vi "Table Load.vi"(8 "error in (no error)":errorcluster, 11 "Work No":refnum<vi>) -> ()   [LabVIEW 2019]
uses:
  Ctrl/Table Save.ctl
  <vilib>/Utility/xml.llb/Read From XML File(string).vi
  LLB/Commonly VI/Main Glb.vi
  <vilib>/Utility/xml.llb/Write to XML File(string).vi
  LLB/Commonly VI.lvlib
panel:
  out "NG數量":string
  out "良品數量":string
  out "工單號碼Table":cluster{"Table Control":string[][]}[](array[cluster])
  out "EnfMeasureTable":cluster{"Table Control":string[][]}[](array[cluster])
  in  "EnfMeasureTable 5":cluster{"Table Control":string[][]}[](array[cluster])
  out "EnfMeasureTable 3":cluster{"Table Control":string[][]}[](array[cluster])
  out "value":cluster{"Table Control":string[][]}[](array[cluster])
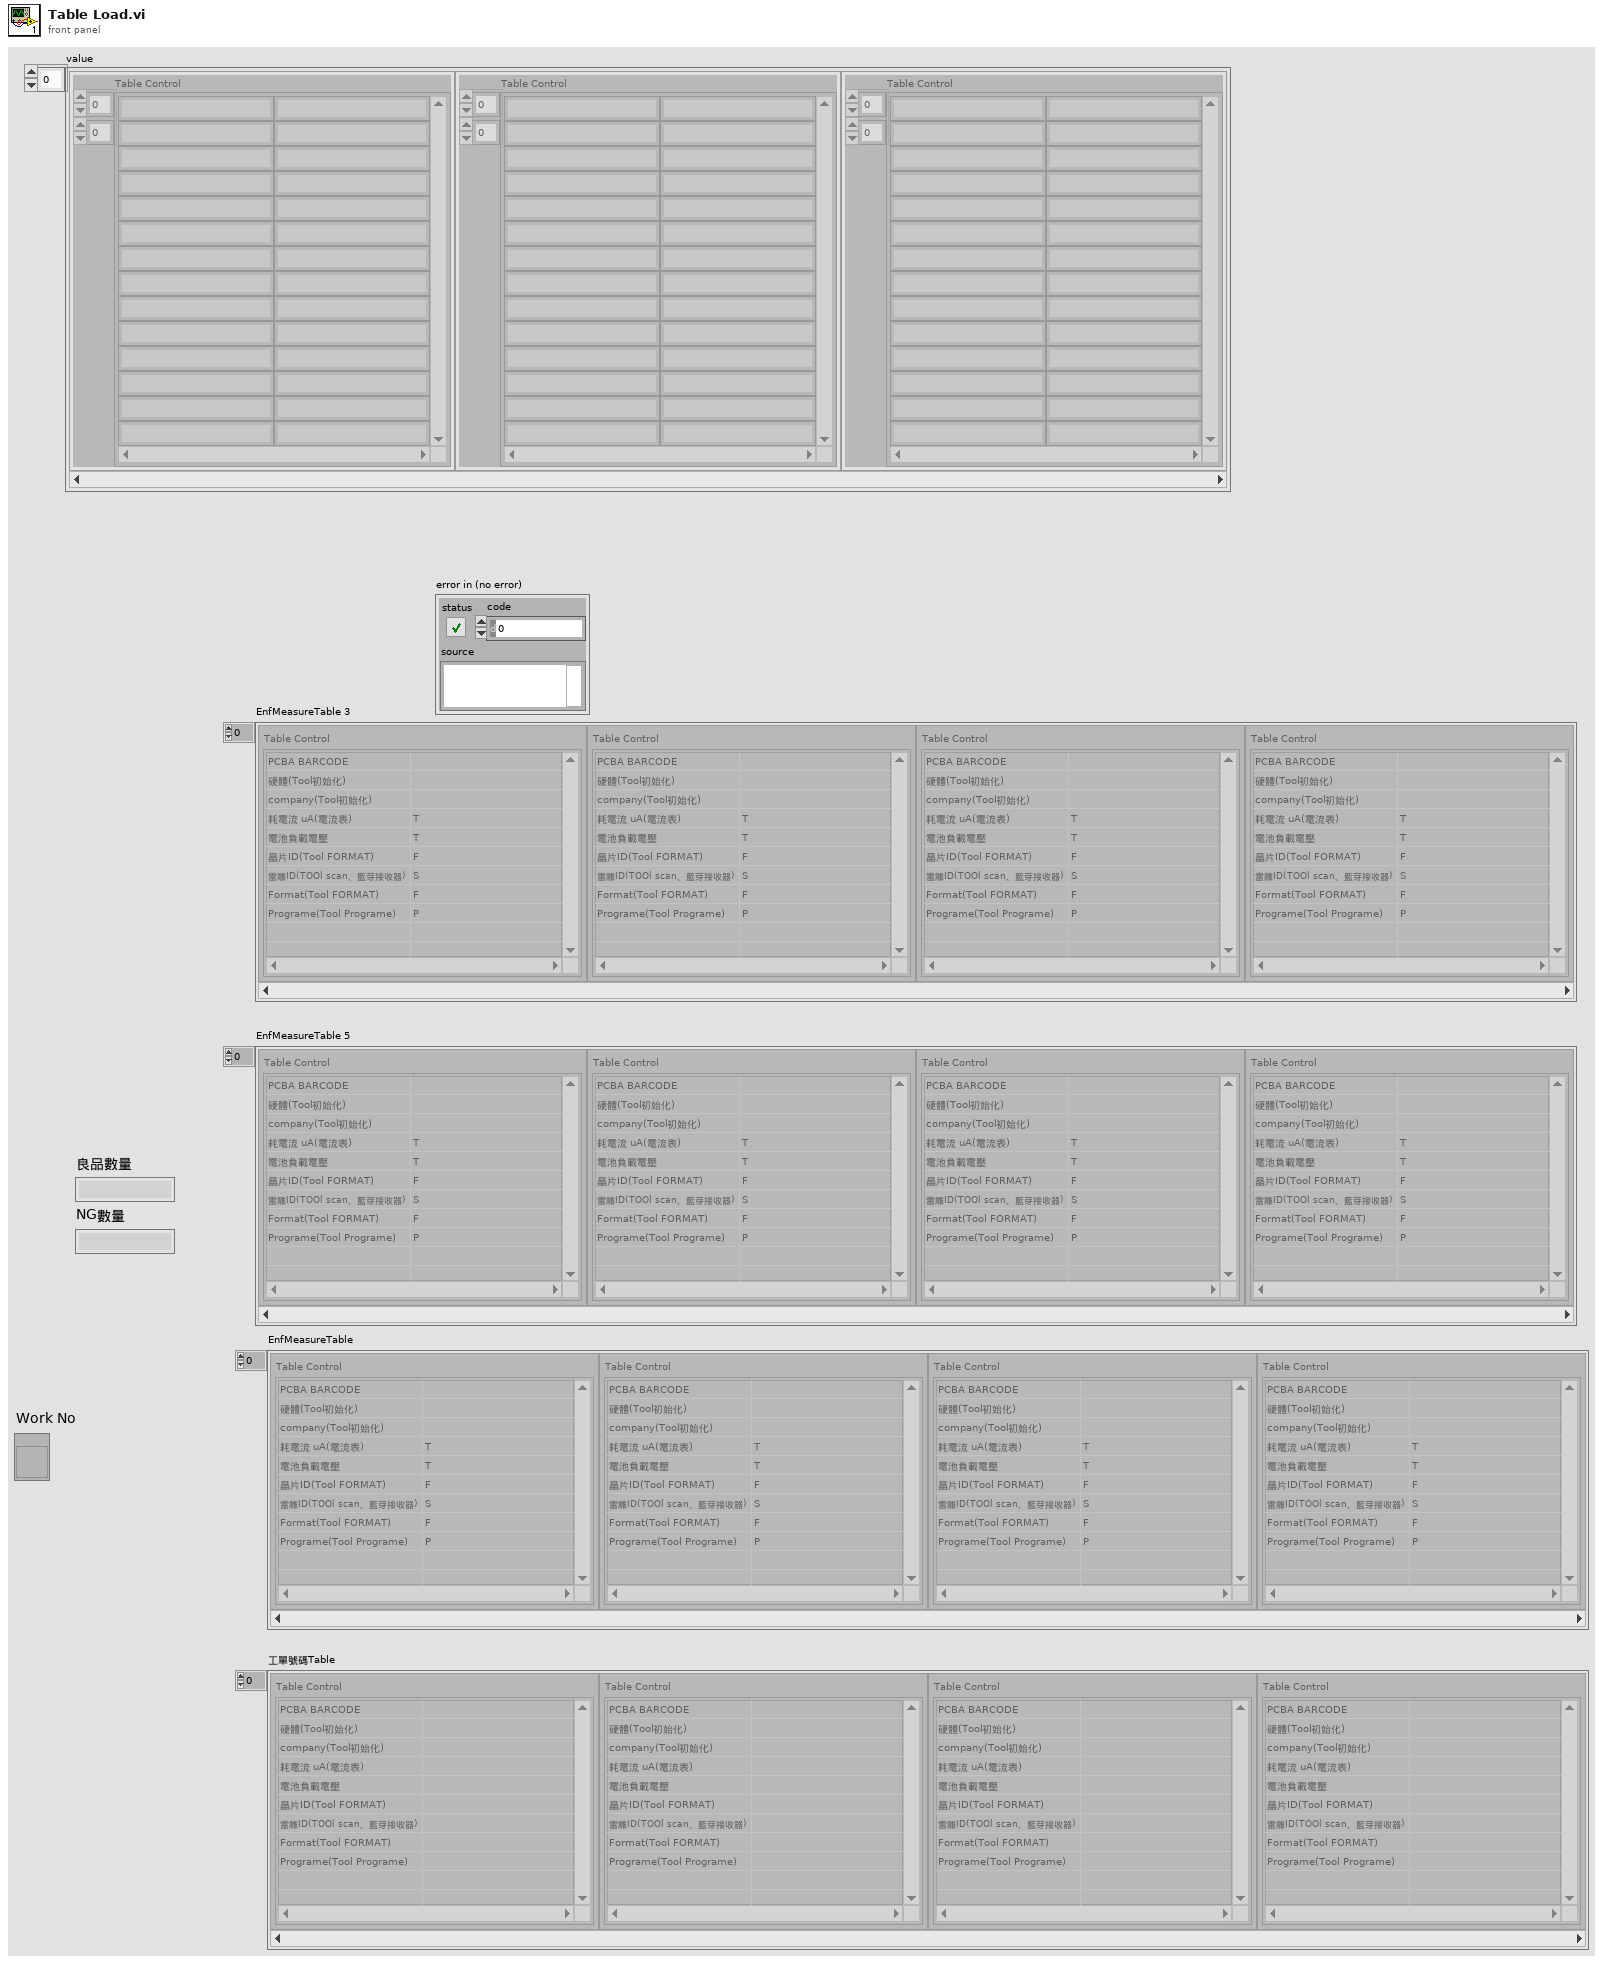
[diagram p1: front panel]
types:
  T1 = typedef "Table Save.ctl" = enum16{"initial", "Add", "Write", "Replace", "Delete", "REad", "RedTable", "Load"}
  T2 = typedef "工單號碼_Index.ctl" = enum16{"工單號碼", "產品料號", "品名", "作業員", "生產總數", "量品數量", "NG數量", "良率%"}
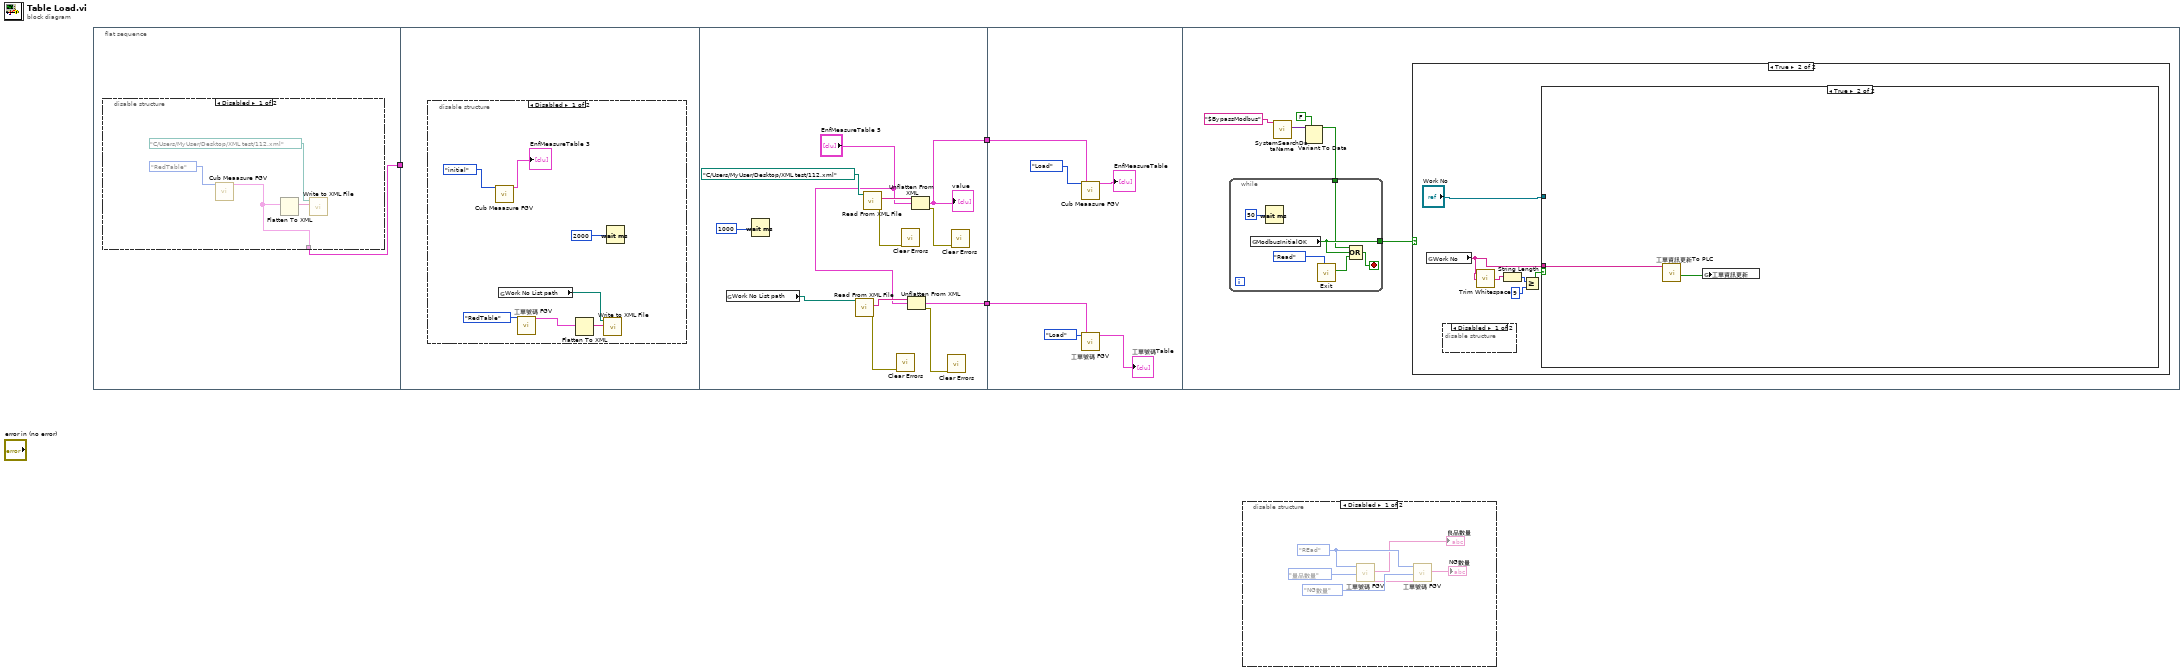
[diagram p0: block diagram]
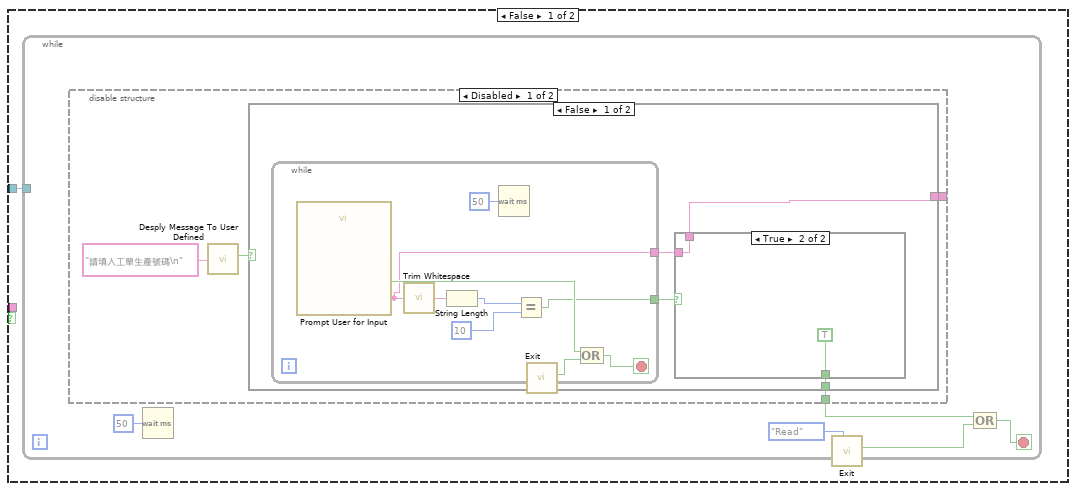
[diagram p6: hidden frame]
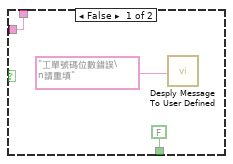
[diagram p7: hidden frame]
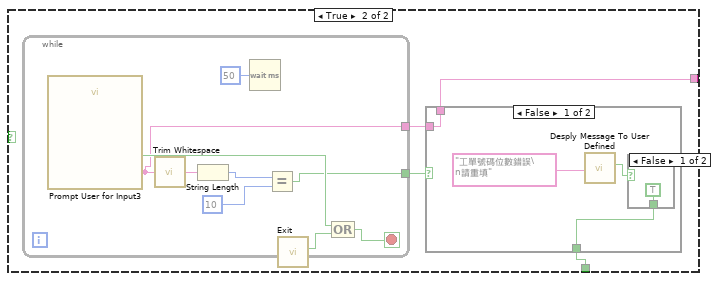
[diagram p8: hidden frame]
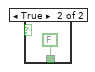
[diagram p9: hidden frame]
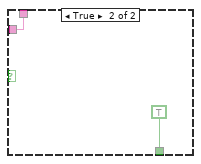
[diagram p10: hidden frame]
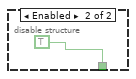
[diagram p11: hidden frame]
diagram:
  n1 = flat-sequence {
    tunnel: [w4] -> w3
    tunnel: w3 -> [_]
    tunnel: [w24] -> w2
    tunnel: [w18] -> w1
    tunnel: w2 -> [w31]
    tunnel: w1 -> [w29]
    frame #0 {
      n2 = disable-structure shown="Disabled" {
        disable-tunnel: [w5 _] -> w4
        frame Disabled {
          n3 = call "Cub Meaasure FGV.vi"("Action"=Table_Save."RedTable") -> ("Total Table"=w5:cluster{"Table Control":string[][]}[])  [unwired: 8 in, 6 out]
          n4 = Flatten To XML(anything=w5) -> (xml string=w8:string)
          n5 = call-poly <vilib>:"Write to XML File.vi"("XML Input"=w8, "XML File Path"=path "C:/Users/MyUser/Desktop/XML test/112.xml") -> ()  [unwired: 7 in, 3 out]
        }
        frame Enabled {
        }
      }
    }
    frame #1 {
      n6 = disable-structure shown="Disabled" {
        frame Disabled {
          n7 = call "Cub Meaasure FGV.vi"("Action"=Table_Save."initial") -> ("Total Table"=→"EnfMeasureTable 3":cluster{"Table Control":string[][]}[])  [unwired: 8 in, 6 out]
          n8 = global read "Main Glb.vi" "Work No List path"() -> (w12:path)
          n9 = call "工單號碼 FGV.vi"("Action"=Table_Save."RedTable") -> ("Total Table"=w10:cluster{"Table Control":string[][]}[])  [unwired: 11 in, 7 out]
          n10 = Flatten To XML(anything=w10) -> (xml string=w11:string)
          n11 = call-poly <vilib>:"Write to XML File.vi"("XML Input"=w11, "XML File Path"=w12) -> ()  [unwired: 7 in, 3 out]
          n12 = Wait (ms)(milliseconds to wait=2000) -> ()  [unwired: 1 out]
        }
        frame Enabled {
        }
      }
    }
    frame #2 {
      n13 = global read "Main Glb.vi" "Work No List path"() -> (w21:path)
      n14 = Wait (ms)(milliseconds to wait=1000) -> ()  [unwired: 1 out]
      n15 = call-poly <vilib>:"Read From XML File.vi"("XML File Path"=w21) -> ("error out"=w20:errorcluster, "XML Elements"=w19:string)  [unwired: 8 in, 1 out]
      n16 = call-poly <vilib>:"Read From XML File.vi"("XML File Path"=path "C:/Users/MyUser/Desktop/XML test/112.xml") -> ("error out"=w22:errorcluster, "XML Elements"=w27:string)  [unwired: 8 in, 1 out]
      n17 = call <vilib>:"Clear Errors.vi"("error in (no error)"=w20) -> ()  [unwired: 5 in, 2 out]
      n18 = call <vilib>:"Clear Errors.vi"("error in (no error)"=w22) -> ()  [unwired: 5 in, 2 out]
      n19 = Unflatten From XML(xml string=w19, type="EnfMeasureTable 5") -> (value=w18:cluster{"Table Control":string[][]}[], error out=w16:errorcluster)  [unwired: 1 in]
      n20 = Unflatten From XML(xml string=w27, type="EnfMeasureTable 5") -> (value=w24:cluster{"Table Control":string[][]}[], error out=w23:errorcluster)  [unwired: 1 in]
      "value" <- w24
      n21 = call <vilib>:"Clear Errors.vi"("error in (no error)"=w16) -> ()  [unwired: 5 in, 2 out]
      n22 = call <vilib>:"Clear Errors.vi"("error in (no error)"=w23) -> ()  [unwired: 5 in, 2 out]
    }
    frame #3 {
      n23 = call "Cub Meaasure FGV.vi"("Action"=Table_Save."Load", "Table Load"=w31) -> ("Total Table"=→"EnfMeasureTable":cluster{"Table Control":string[][]}[])  [unwired: 10 in, 7 out]
      n24 = call "工單號碼 FGV.vi"("Action"=Table_Save."Load", "Table Load"=w29) -> ("Total Table"=→"工單號碼Table":cluster{"Table Control":string[][]}[])  [unwired: 10 in, 7 out]
    }
    frame #4 {
      n25 = call "SystemSearchDataName.vi"("element"="$BypassModbus") -> ("variant"=w37:variant)  [unwired: 8 in, 2 out]
      n26 = Variant To Data(type=FALSE, Variant=w37) -> (data=w34:bool)  [unwired: 1 in, 1 out]
      n27 = while {
        tunnel: [w99] -> w38
        tunnel: w34 -> [w97]
        stop <- w100 stop-if-true
        n28 = global read "Main Glb.vi" "ModbusInitialOK"() -> (w99:bool)
        n29 = Wait (ms)(milliseconds to wait=50) -> ()  [unwired: 1 out]
        n30 = call "Exit.vi"("Enum"=enum16{"Initial", "Read", "Write"}."Read") -> ("ExitOut"=w101:bool)  [unwired: 10 in]
        n31 = Compound Arithmetic op=OR(w97, w99, w101) -> (w100:bool)
      }
      n32 = case shown="True" w38 {
        frame False {
        }
        frame True {
          n33 = global read "Main Glb.vi" "Work No"() -> (w40:string)
          n34 = disable-structure shown="Disabled" {
            frame Disabled {
            }
            frame Enabled {
            }
          }
          n35 = call <vilib>:"Trim Whitespace.vi"("string"=w40) -> ("trimmed string"=w39:string)  [unwired: 1 in]
          n36 = String Length(string=w39) -> (length=w44:i32)
          n37 = Greater Or Equal?(x=w44, y=9) -> (x >= y?=w42:bool)
          n38 = case shown="True" w42 {
            tunnel: w40 -> [_ w96]
            tunnel: "Work No" -> [w45 _]
            frame False {
              n39 = while {
                tunnel: w45 -> [_]
                stop <- w46 stop-if-true
                n40 = disable-structure shown="Disabled" {
                  disable-tunnel: [w52 TRUE] -> w49
                  disable-tunnel: [w51 _] -> _
                  frame Disabled {
                    n41 = call "Desply Message To User Defined.vi"("Message"="請填入工單生產號碼\n") -> ("關閉/Close"=w53:bool)  [unwired: 9 in, 1 out]
                    n42 = case shown="False" w53 {
                      tunnel: [w56 w74] -> w51
                      tunnel: [w55 w73] -> w52
                      frame False {
                        n43 = while {
                          tunnel: [w66] -> w58
                          tunnel: [w65] -> w57
                          stop <- w68 stop-if-true
                          n44 = call "Prompt User for Input"() -> ("Work No"=w65:string, "OK"=w67:bool)  [unwired: 17 in, 1 out]
                          n45 = call <vilib>:"Trim Whitespace.vi"("string"=w65) -> ("trimmed string"=w72:string)  [unwired: 1 in]
                          n46 = String Length(string=w72) -> (length=w71:i32)
                          n47 = Wait (ms)(milliseconds to wait=u32 50) -> ()  [unwired: 1 out]
                          n48 = Equal?(x=w71, y=10) -> (x = y?=w66:bool)
                          n49 = call "Exit.vi"() -> ("ExitOut"=w69:bool)  [unwired: 11 in]
                          n50 = Compound Arithmetic op=OR(w67, w69) -> (w68:bool)
                        }
                        n51 = case shown="True" w58 {
                          tunnel: w57 -> [w61 w63]
                          tunnel: [w61 w63] -> w56
                          tunnel: [FALSE TRUE] -> w55
                          frame False {
                            n52 = call "Desply Message To User Defined.vi"("Message"="工單號碼位數錯誤\n請重填") -> ()  [unwired: 9 in, 2 out]
                          }
                          frame True {
                          }
                        }
                      }
                      frame True {
                        n53 = while {
                          tunnel: [w87] -> w76
                          tunnel: [w86] -> w75
                          stop <- w89 stop-if-true
                          n54 = call "Prompt User for Input3"() -> ("Work No"=w86:string, "OK"=w88:bool)  [unwired: 17 in, 1 out]
                          n55 = call <vilib>:"Trim Whitespace.vi"("string"=w86) -> ("trimmed string"=w93:string)  [unwired: 1 in]
                          n56 = String Length(string=w93) -> (length=w92:i32)
                          n57 = Wait (ms)(milliseconds to wait=u32 50) -> ()  [unwired: 1 out]
                          n58 = Equal?(x=w92, y=10) -> (x = y?=w87:bool)
                          n59 = call "Exit.vi"() -> ("ExitOut"=w90:bool)  [unwired: 11 in]
                          n60 = Compound Arithmetic op=OR(w88, w90) -> (w89:bool)
                        }
                        n61 = case shown="False" w76 {
                          tunnel: w75 -> [w80 w84]
                          tunnel: [w80 w84] -> w74
                          tunnel: [w78 TRUE] -> w73
                          frame False {
                            n62 = call "Desply Message To User Defined.vi"("Message"="工單號碼位數錯誤\n請重填") -> ("關閉/Close"=w77:bool)  [unwired: 9 in, 1 out]
                            n63 = case shown="False" w77 {
                              tunnel: [TRUE FALSE] -> w78
                              frame False {
                              }
                              frame True {
                              }
                            }
                          }
                          frame True {
                          }
                        }
                      }
                    }
                  }
                  frame Enabled {
                  }
                }
                n64 = Wait (ms)(milliseconds to wait=u32 50) -> ()  [unwired: 1 out]
                n65 = call "Exit.vi"("Enum"=enum16{"Initial", "Read", "Write"}."Read") -> ("ExitOut"=w48:bool)  [unwired: 10 in]
                n66 = Compound Arithmetic op=OR(w49, w48) -> (w46:bool)
              }
            }
            frame True {
              n67 = call "工單資訊更新To PLC.vi"("Work No"=w96) -> ("Boolean"=w95:bool)  [unwired: 7 in, 3 out]
              n68 = global write "Main Glb.vi" "工單資訊更新"(w95) -> ()
            }
          }
        }
      }
    }
  }
  n69 = disable-structure shown="Disabled" {
    frame Disabled {
      w107 = Table_Save."REad" ("Action")
      n70 = call "工單號碼 FGV.vi"("Action"=w107, "工單Data Save Index"=工單號碼_Index."NG數量" ("工單號碼Index")) -> ("工單號碼"=w105:string, "Read Index Data"=→"NG數量":string)  [unwired: 9 in, 7 out]
      n71 = call "工單號碼 FGV.vi"("Action"=w107, "工單Data Save Index"=工單號碼_Index."量品數量" ("工單號碼Index"), "工單號碼"=w105) -> ("Read Index Data"=→"良品數量":string)  [unwired: 9 in, 7 out]
    }
    frame Enabled {
    }
  }
